vi "set_org.vi"(2 "error in (no error)":errorcluster caption="错误输入（无错误）", 3 "pos":dbl, 4 "OneMotion 输入":refnum<class "OneMotion.lvclass">) -> (0 "error out":errorcluster caption="错误输出", 1 "OneMotion 输出":refnum<class "OneMotion.lvclass">)   [LabVIEW 2016, in "MotionControl_UFO_3DOF.lvlib" / "OneMotion.lvclass"]
uses:
  <userlib>/MotionControl_UFO_3DOF/OneMotion/OneMotion.lvclass
  <userlib>/MotionControl_UFO_3DOF/OneMotion/OneMotion.lvclass/OneMotion.ctl
  <userlib>/MotionControl_UFO_3DOF/StepMotor/StepMotor.lvclass
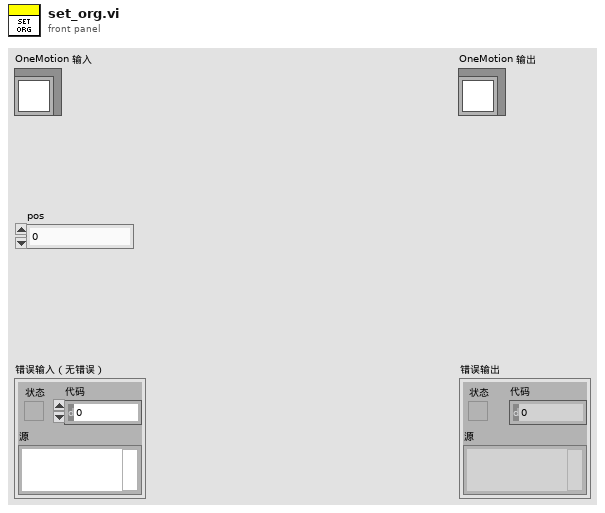
[diagram p1: front panel]
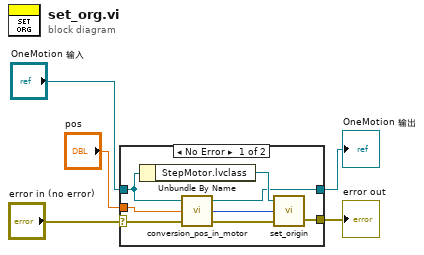
[diagram p0: block diagram]
diagram:
  n1 = case shown="No Error" "error in (no error)" {
    selector: "error in (no error)" -> [w8 w15]
    tunnel: [w12 w15] -> w4
    tunnel: [w7 w14] -> w2
    tunnel: "OneMotion 输入" -> [w9 w14]
    tunnel: "pos" -> [w11 _]
    frame No Error {
      n2 = Unbundle By Name(w9) -> ("StepMotor.lvclass"=w13:refnum<class "StepMotor.lvclass">)
      n3 = call <userlib>:"conversion_pos_in_motor.vi"("error in (no error)"=w8, "pos"=w11, "OneMotion 输入"=w9) -> ("error out"=w6:errorcluster, "pos in motor"=w10:i32, "OneMotion 输出"=w7:refnum<class "OneMotion.lvclass">)
      n4 = call <userlib>:"set_origin.vi"("error in (no error)"=w6, "value"=w10, "StepMotor输入"=w13) -> ("error out"=w12:errorcluster)  [unwired: 1 out]
    }
    frame Error {
    }
  }
  "error out" <- w4
  "OneMotion 输出" <- w2
